vi "run.vi"(5 "RunGlobalTearDown":bool, 7 "RunGlobalSetup":bool, 8 "error in (no error)":errorcluster, 10 "TestResult in (None: Create New)":refnum<class "TestResult.lvclass">, 11 "TestCase in":refnum<class "TestCase.lvclass">) -> (0 "error out":errorcluster, 2 "TestResult out":refnum<class "TestResult.lvclass">, 3 "TestCase out":refnum<class "TestCase.lvclass">)   [LabVIEW 2013, in "TestCase.lvclass"]
uses:
  TestCase.lvclass
  TestResult/TestResult.lvclass
  TestCase.lvclass/TestCase.ctl
  private/method--Enum.ctl
  JKI Reuse/Is an Error (error cluster)__jki_lib_error_handling -- VI Tester.vi
  Libraries/VITesterUtilities.lvlib
panel:
  # "JKI VI Tester for LabVIEW\nhttp://jkisoft.com/vi-tester\nCopyright (C) 2007-2009, JKI <info@jkisoft.com>\nALL RIGHTS RESERVED"
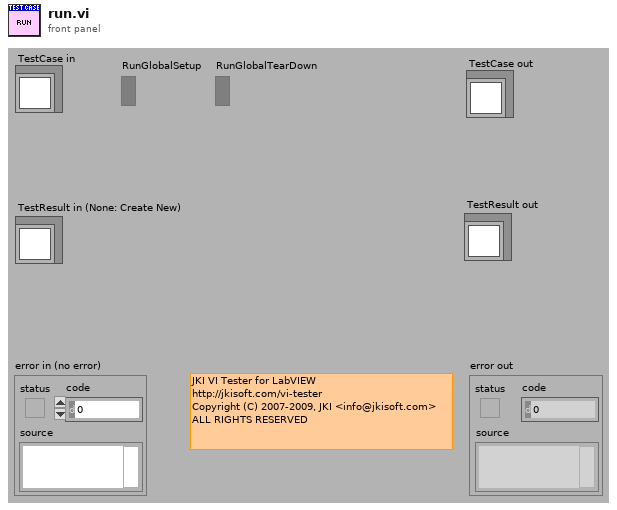
[diagram p1: front panel]
types:
  T1 = typedef "TestCase.lvclass/method--Enum.ctl" = enum16{"setUp", "testMethod", "tearDown"}
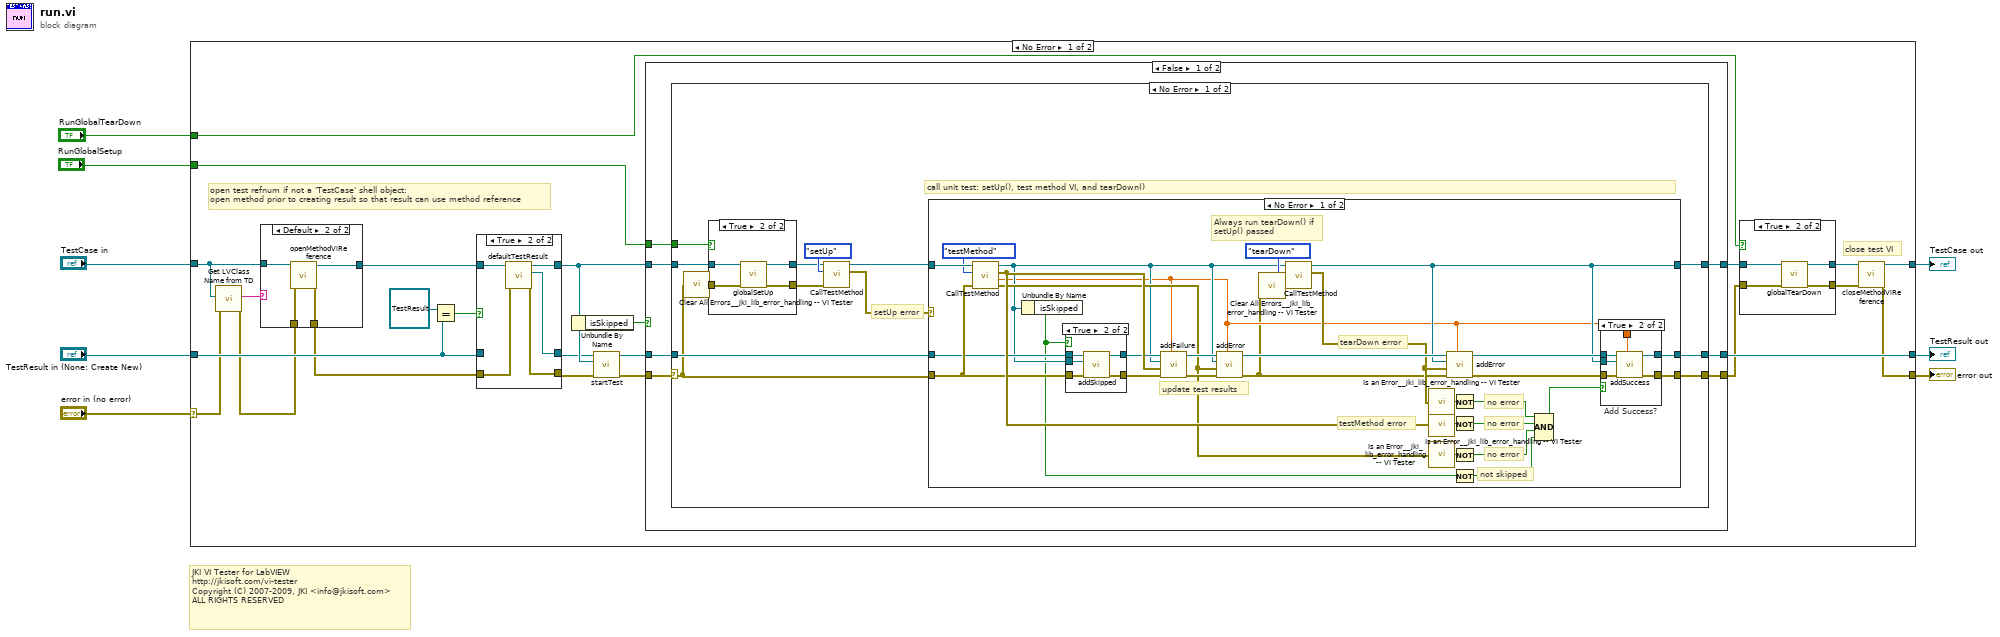
[diagram p0: block diagram]
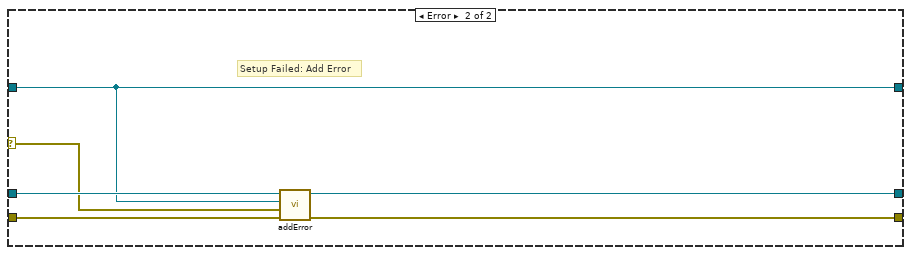
[diagram p7: hidden frame]
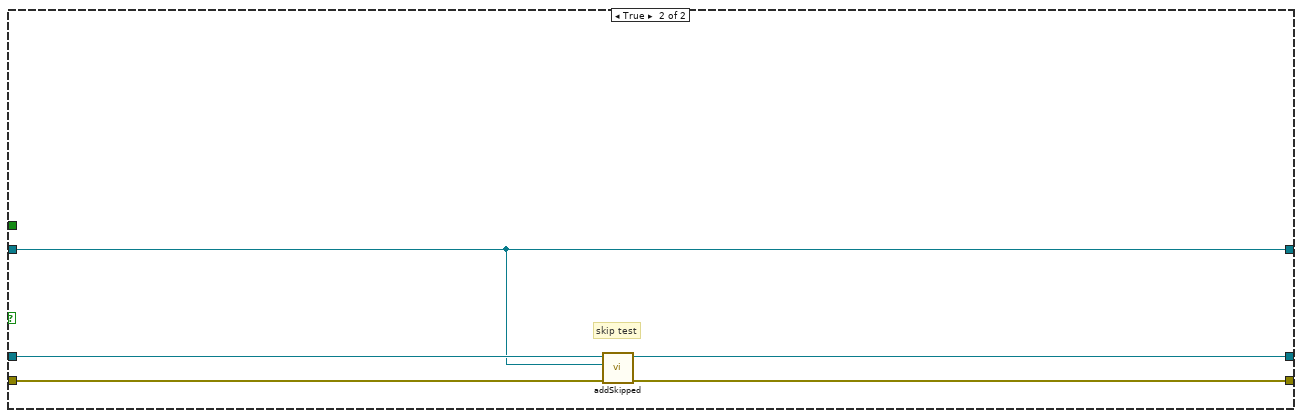
[diagram p9: hidden frame]
diagram:
  # "JKI VI Tester for LabVIEW\nhttp://jkisoft.com/vi-tester\nCopyright (C) 2007-2009, JKI <info@jkisoft.com>\nALL RIGHTS RESERVED"
  n1 = case shown="No Error" "error in (no error)" {
    selector: "error in (no error)" -> [w16 w141]
    tunnel: [w18 w141] -> w7
    tunnel: [w19 w140] -> w5
    tunnel: "TestCase in" -> [w17 w140]
    tunnel: "TestResult in (None: Create New)" -> [w30 w139]
    tunnel: [w29 w139] -> w3
    tunnel: "RunGlobalSetup" -> [w14 _]
    tunnel: "RunGlobalTearDown" -> [w9 _]
    frame No Error {
      # "close test VI"
      # "open test refnum if not a 'TestCase' shell object:\nopen method prior to creating result so that result can use method reference"
      n2 = call "Get LVClass Name from TD.vi"("error in"=w16, "Variant"=w17) -> ("error out"=w15:errorcluster, "LVClass Name"=w22:string)  [unwired: 8 in]
      n3 = case shown="Default" w22 {
        tunnel: w15 -> [w39 w44]
        tunnel: [w40 w43] -> w20
        tunnel: [w39 w42] -> w21
        tunnel: w17 -> [w40 w41]
        frame "TestCase.lvclass" {
        }
        frame Default {
          n4 = call "openMethodViReference.vi"("error in (no error)"=w44, "TestCase in"=w41) -> ("error out"=w42:errorcluster, "TestCase out"=w43:refnum<class "TestCase.lvclass">)  [unwired: 8 in]
        }
      }
      n5 = Equal?(x=refnum<class "TestResult.lvclass"> refnum ("result (None: Create New)"), y=w30) -> (x = y?=w31:bool)
      n6 = case shown="True" w31 {
        tunnel: w20 -> [w133 w138]
        tunnel: [w133 w137] -> w27
        tunnel: [w132 w136] -> w24
        tunnel: w30 -> [w132 _]
        tunnel: w21 -> [w131 w135]
        tunnel: [w131 w134] -> w25
        frame False {
        }
        frame True {
          n7 = call-dynamic "defaultTestResult.vi"("error in (no error)"=w135, "TestCase in"=w138) -> ("error out"=w134:errorcluster, "TestResult"=w136:refnum<class "TestResult.lvclass">, "TestCase out"=w137:refnum<class "TestCase.lvclass">)  [unwired: 7 in]
        }
      }
      n8 = Unbundle By Name(w27) -> ("isSkipped"=w28:bool)
      n9 = call-dynamic "startTest.vi"("error in (no error)"=w25, "test"=w27, "TestResult in"=w24) -> ("error out"=w26:errorcluster, "TestResult in"=w23:refnum<class "TestResult.lvclass">)  [unwired: 7 in]
      n10 = case shown="False" w28 {
        tunnel: w23 -> [w49 w130]
        tunnel: w26 -> [w48 w129]
        tunnel: [w46 w126] -> w13
        tunnel: [w47 w128] -> w11
        tunnel: [w51 w127] -> w29
        tunnel: w27 -> [w50 w126]
        tunnel: w14 -> [w45 _]
        frame False {
          n11 = case shown="No Error" w48 {
            selector: w48 -> [w57 w124]
            tunnel: w50 -> [w54 w125]
            tunnel: [w62 w125] -> w46
            tunnel: w49 -> [w64 w123]
            tunnel: [w63 w124] -> w47
            tunnel: [w61 w123] -> w51
            tunnel: w45 -> [w52 _]
            frame No Error {
              # "setUp error"
              # "call unit test: setUp(), test method VI, and tearDown()"
              n12 = call "Clear All Errors__jki_lib_error_handling -- VI Tester.vi"("error in"=w57) -> ("no error out"=w56:errorcluster)  [unwired: 4 in]
              n13 = case shown="True" w52 {
                tunnel: w56 -> [w65 w69]
                tunnel: [w65 w68] -> w55
                tunnel: w54 -> [w66 w70]
                tunnel: [w66 w67] -> w53
                frame False {
                }
                frame True {
                  n14 = call-dynamic "globalSetUp.vi"("error in (no error)"=w69, "TestCase in"=w70) -> ("error out"=w68:errorcluster, "TestCase out"=w67:refnum<class "TestCase.lvclass">)  [unwired: 8 in]
                }
              }
              n15 = call "CallTestMethod.vi"("error in"=w55, "method"=method--Enum."setUp", "TestCase in"=w53) -> ("Test Method Error"=w58:errorcluster, "TestCase out"=w59:refnum<class "TestCase.lvclass">)  [unwired: 5 in, 2 out]
              n16 = case shown="No Error" w58 {
                selector: w58 -> [_ w120]
                tunnel: w64 -> [w77 w122]
                tunnel: w57 -> [w79 w121]
                tunnel: [w94 w118] -> w63
                tunnel: w59 -> [w91 w119]
                tunnel: [w83 w119] -> w62
                tunnel: [w92 w117] -> w61
                frame No Error {
                  # "not skipped"
                  # "no error"
                  # "testMethod error"
                  # "tearDown error"
                  # "no error"
                  # "no error"
                  # "update test results"
                  # "Always run tearDown() if setUp() passed"
                  n17 = call "CallTestMethod.vi"("error in"=w79, "method"=method--Enum."testMethod", "TestCase in"=w91) -> ("error out"=w81:errorcluster, "execution time (sec)"=w72:dbl, "Test Method Error"=w88:errorcluster, "TestCase out"=w75:refnum<class "TestCase.lvclass">)  [unwired: 5 in]
                  n18 = Unbundle By Name(w75) -> ("isSkipped"=w74:bool)
                  n19 = case shown="True" w74 {
                    tunnel: w79 -> [w102 w108]
                    tunnel: [w102 w107] -> w78
                    tunnel: w77 -> [w103 w106]
                    tunnel: [w103 w105] -> w76
                    tunnel: w75 -> [_ w104]
                    frame False {
                    }
                    frame True {
                      n20 = call-dynamic "addSkipped.vi"("error in (no error)"=w108, "test"=w104, "TestResult in"=w106) -> ("error out"=w107:errorcluster, "TestResult out"=w105:refnum<class "TestResult.lvclass">)  [unwired: 7 in]
                    }
                  }
                  n21 = call-dynamic "addFailure.vi"("execution time (sec)"=w72, "error in (no error)"=w78, "test error"=w88, "test"=w75, "TestResult in"=w76) -> ("error out"=w90:errorcluster, "TestResult out"=w101:refnum<class "TestResult.lvclass">)  [unwired: 5 in]
                  n22 = call-dynamic "addError.vi"("execution time (sec)"=w72, "error in (no error)"=w90, "test error"=w81, "test"=w75, "TestResult in"=w101) -> ("error out"=w71:errorcluster, "TestResult out"=w100:refnum<class "TestResult.lvclass">)  [unwired: 5 in]
                  n23 = call "Clear All Errors__jki_lib_error_handling -- VI Tester.vi"("error in"=w71) -> ("no error out"=w86:errorcluster)  [unwired: 4 in]
                  n24 = call "CallTestMethod.vi"("error in"=w86, "method"=method--Enum."tearDown", "TestCase in"=w75) -> ("Test Method Error"=w84:errorcluster, "TestCase out"=w83:refnum<class "TestCase.lvclass">)  [unwired: 5 in, 2 out]
                  n25 = call-poly "Is an Error__jki_lib_error_handling -- VI Tester.vi"("error in"=w84) -> ("error?"=w99:bool)  [unwired: 8 in]
                  n26 = call-poly "Is an Error__jki_lib_error_handling -- VI Tester.vi"("error in"=w88) -> ("error?"=w89:bool)  [unwired: 8 in]
                  n27 = call-poly "Is an Error__jki_lib_error_handling -- VI Tester.vi"("error in"=w81) -> ("error?"=w82:bool)  [unwired: 8 in]
                  n28 = call-dynamic "addError.vi"("execution time (sec)"=w72, "error in (no error)"=w71, "test error"=w84, "test"=w83, "TestResult in"=w100) -> ("error out"=w95:errorcluster, "TestResult out"=w96:refnum<class "TestResult.lvclass">)  [unwired: 5 in]
                  n29 = Not(x=w99) -> (.not. x?=w98:bool)
                  n30 = Not(x=w89) -> (.not. x?=w97:bool)
                  n31 = Not(x=w82) -> (.not. x?=w80:bool)
                  n32 = Not(x=w74) -> (.not. x?=w73:bool)
                  n33 = Compound Arithmetic op=AND(w98, w97, w80, w73) -> (w93:bool)
                  n34 = case "Add Success?" shown="True" w93 {
                    tunnel: w96 -> [w110 w116]
                    tunnel: w95 -> [w109 w115]
                    tunnel: [w109 w114] -> w94
                    tunnel: [w110 w113] -> w92
                    tunnel: w83 -> [_ w112]
                    tunnel: w72 -> [_ w111]
                    frame False {
                    }
                    frame True {
                      n35 = call-dynamic "addSuccess.vi"("execution time (sec)"=w111, "error in (no error)"=w115, "test"=w112, "TestResult in"=w116) -> ("error out"=w114:errorcluster, "TestResult in"=w113:refnum<class "TestResult.lvclass">)  [unwired: 6 in]
                    }
                  }
                }
                frame Error {
                  # "Setup Failed: Add Error"
                  n36 = call-dynamic "addError.vi"("error in (no error)"=w121, "test error"=w120, "test"=w119, "TestResult in"=w122) -> ("error out"=w118:errorcluster, "TestResult out"=w117:refnum<class "TestResult.lvclass">)  [unwired: 6 in]
                }
              }
            }
            frame Error {
            }
          }
        }
        frame True {
          # "skip test"
          n37 = call-dynamic "addSkipped.vi"("error in (no error)"=w129, "test"=w126, "TestResult in"=w130) -> ("error out"=w128:errorcluster, "TestResult out"=w127:refnum<class "TestResult.lvclass">)  [unwired: 7 in]
        }
      }
      n38 = case shown="True" w9 {
        tunnel: w11 -> [w33 w37]
        tunnel: [w33 w35] -> w10
        tunnel: w13 -> [w34 w38]
        tunnel: [w34 w36] -> w12
        frame False {
        }
        frame True {
          n39 = call-dynamic "globalTearDown.vi"("error in (no error)"=w37, "TestCase in"=w38) -> ("error out"=w35:errorcluster, "TestCase out"=w36:refnum<class "TestCase.lvclass">)  [unwired: 8 in]
        }
      }
      n40 = call "closeMethodViReference.vi"("error in (no error)"=w10, "TestCase in"=w12) -> ("error out"=w18:errorcluster, "TestCase in"=w19:refnum<class "TestCase.lvclass">)  [unwired: 8 in]
    }
    frame Error {
    }
  }
  "error out" <- w7
  "TestCase out" <- w5
  "TestResult out" <- w3
